vi "PH_AxisGUI_BaseClass.get Address by Number.vi"(0 "VI in":refnum<vi>, 2 "Axis":i32=-1, 5 "error in (no error)":errorcluster) -> (11 "Axis exists?":bool, 14 "VI out":refnum<vi>, 16 "Address":T1, 17 "Axis exists and is not moving?":bool, 19 "error out":errorcluster)   [LabVIEW 2014, in "PH_AxisGUI_BaseClass.lvlib"]
doc: "This VI gets the Address (Instance and Motor Number) of an Axis; it thereby checks whether the Axis is in the list, the Instance is not empty or \"N/A\" and the axis is not moving."
uses:
  PH_AxisGUI_BaseClass.lvlib
  PH_Stepmotor_BaseClass/PH_Stepmotor_BaseClass.Axis Address.ctl
  PH_Stepmotor_BaseClass/PH_Stepmotor_BaseClass.lvlib
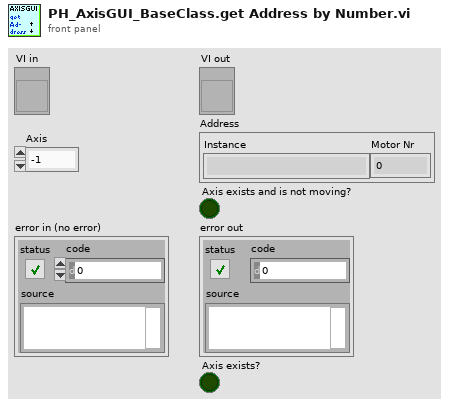
[diagram p1: front panel]
types:
  T1 = typedef "PH_Stepmotor_BaseClass.lvlib/PH_Stepmotor_BaseClass.Axis Address.ctl" = cluster{"Instance":string, "Motor Nr":i32}
  T2 = typedef "PH_AxisGUI_BaseClass.lvlib/PH_AxisGUI_BaseClass.i attribute.ctl" = cluster{"Axes":T3[]}
  T3 = typedef "PH_AxisGUI_BaseClass.lvlib/PH_AxisGUI_BaseClass.Axis Attributes.ctl" = cluster{"Axis GUI Refs":T4, "Address":T1, "Name":string, "Label \"Back\"":string, "Labell \"Forth\"":string, "Moving?":bool}
  T4 = typedef "PH_AxisGUI_BaseClass.lvlib/PH_AxisGUI_BaseClass.Axis GUI Refs.ctl" = cluster{"Back":refnum<vi>, "Forth":refnum<vi>, "Status":refnum<vi>, "Target":refnum<vi>, "Address":refnum<vi>, "Status Bar":refnum<vi>, "Settings":refnum<vi>, "Activity":refnum<vi>, "Clear Error":refnum<vi>}
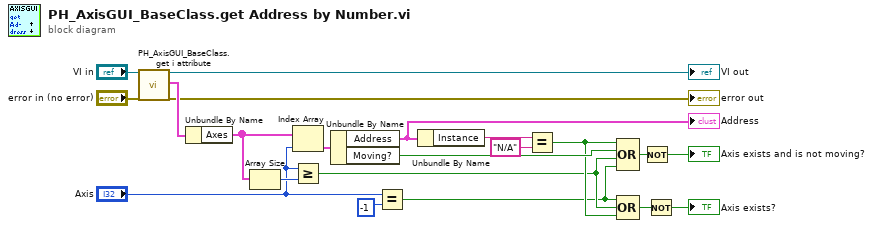
[diagram p0: block diagram]
diagram:
  n1 = call "PH_AxisGUI_BaseClass.get i attribute.vi"("i ref in"="VI in", "error in (no error)"="error in (no error)") -> ("i ref out"=→"VI out":refnum<vi>, "i attribute"=w11:T2, "error out"=→"error out":errorcluster)  [unwired: 15 in]
  n2 = Unbundle By Name(w11) -> ("Axes"=w12:T3[])
  n3 = Array Size(array=w12) -> (size(s)=w13:i32)
  n4 = Index Array(array=w12, index="Axis") -> (element=w17:T3)
  n5 = Greater Or Equal?(x="Axis", y=w13) -> (x >= y?=w4:bool)
  n6 = Unbundle By Name(w17) -> ("Address"=w16:T1, "Moving?"=w20:bool)
  "Address" <- w16
  n7 = Equal?(x="Axis", y=-1) -> (x = y?=w3:bool)
  n8 = Unbundle By Name(w16) -> ("Instance"=w18:string)
  n9 = Equal?(x=w18, y="N/A") -> (x = y?=w5:bool)
  n10 = Compound Arithmetic op=OR(w5, w20, w4, w3) -> (w21:bool)
  n11 = Compound Arithmetic op=OR(w3, w4, w5) -> (w2:bool)
  n12 = Not(x=w21) -> (.not. x?=→"Axis exists and is not moving?":bool)
  n13 = Not(x=w2) -> (.not. x?=→"Axis exists?":bool)
